vi "Initialize.vi"(8 "error in":errorcluster, 11 "Plugin in":refnum<class "Performanced XNET CAN Logger.lvclass">) -> (0 "error out":errorcluster, 3 "Plugin out":refnum<class "Performanced XNET CAN Logger.lvclass">)   [LabVIEW 2021, in "Performanced XNET CAN Logger.lvlib" / "Performanced XNET CAN Logger.lvclass"]
uses:
  Performanced XNET CAN Logger.lvclass
  C:/Program Files/National Instruments/LabVIEW 2021/vi.lib/FlexLogger/SDK/PluginSDK.lvlibp/PEFClasses/SDK/Plugin/Plugin.lvclass
  Typedef/Def-CAN Port Configuration.ctl
  Typedef/Def-Data Queue Type.ctl
  Typedef/Def-LogSpec.ctl
  Typedef/Def-Executor Command.ctl
  ForFLPlugin/Def-ExecutorConfigurations.ctl
  Performanced XNET CAN Logger.lvclass/Performanced XNET CAN Logger.ctl
  <vilib>/FlexLogger/SDK/PluginSDK.lvlibp/PEFClasses/SDK/Processing Element/Timing Parameters.ctl
  <vilib>/FlexLogger/SDK/PluginSDK.lvlibp/PEFClasses/SDK/Processing Element/Timing Method.ctl
  SubVIs/Global Variables.vi
  <vilib>/FlexLogger/SDK/PluginSDK.lvlibp/PEFClasses/SDK/Plugin/ParameterAccess/Read String.vi
  <vilib>/FlexLogger/SDK/PluginSDK.lvlibp/PEFClasses/SDK/Plugin/ParameterAccess/Write String.vi
  <vilib>/FlexLogger/SDK/PluginSDK.lvlibp/PEFClasses/SDK/Plugin/ParameterAccess/Write Command.vi
  <vilib>/FlexLogger/SDK/PluginSDK.lvlibp/PEFClasses/SDK/Plugin/Plugin.lvclass
  XNET-CAN-Signal-Logger.lvlib
  <vilib>/FlexLogger/SDK/PluginSDK.lvlibp/PEFClasses/SDK/Processing Element/Processing Element.lvclass
  C:/Program Files/National Instruments/LabVIEW 2021/vi.lib/FlexLogger/SDK/PluginSDK.lvlibp/PEFClasses/SDK/Processing Element/Processing Element.lvclass
  C:/Users/NI/Desktop/NIO DongZulong FlexLogger XNET/XNET-CAN-Signal-Logger/src/FlexLogger Plugin/Performanced XNET CAN Logger.lvclass
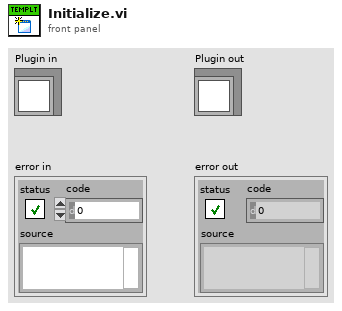
[diagram p1: front panel]
types:
  T1 = typedef "XNET-CAN-Signal-Logger.lvlib/Def-ExecutorConfigurations.ctl" = cluster{"LogSpec":T2, "CAN Configurations":T3[]}
  T2 = typedef "XNET-CAN-Signal-Logger.lvlib/Def-LogSpec.ctl" = cluster{"Log file folder":path, "Log file name":string, "Segment Files":bool, "Segment File Size":i64}
  T3 = typedef "XNET-CAN-Signal-Logger.lvlib/Def-CAN Port Configuration.ctl" = cluster{"CAN Interface":refnum<k21>, "XNET Cluster":refnum<k21>, "#Signals":i32, "Sample Rate (Hz)":dbl}
  T4 = typedef "XNET-CAN-Signal-Logger.lvlib/Def-Executor Command.ctl" = cluster{"Command":string, "Data":variant}
  T5 = typedef "XNET-CAN-Signal-Logger.lvlib/Def-Data Queue Type.ctl" = cluster{"PackageID":i32, "Data":waveform(dbl)[]}
  T6 = typedef "PluginSDK.lvlibp/Processing Element.lvclass/Timing Parameters.ctl" = cluster{"Timing Method":T7, "Timing Period (ms)":i32}
  T7 = typedef "PluginSDK.lvlibp/Processing Element.lvclass/Timing Method.ctl" = enum16{"Periodic", "Immediate", "On Data Ready", "Triggered"}
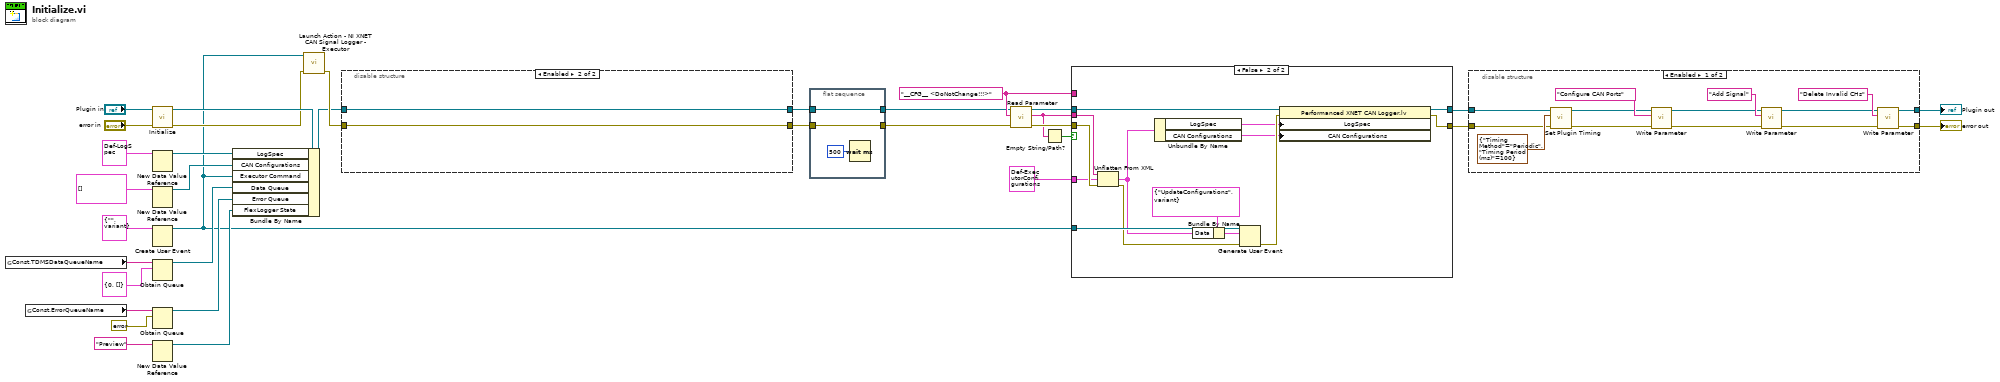
[diagram p0: block diagram]
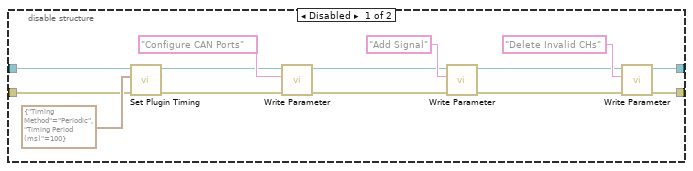
[diagram p3: hidden frame]
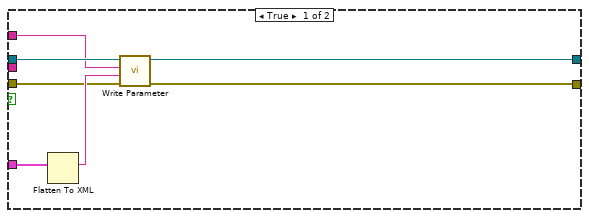
[diagram p4: hidden frame]
diagram:
  w14 = "__CFG__ <DoNotChange!!!>" ("Name")
  n1 = global read "Global Variables.vi" "Const.TDMSDataQueueName"() -> (w29:string)
  n2 = global read "Global Variables.vi" "Const.ErrorQueueName"() -> (w23:string)
  n3 = call-parent "Initialize.vi"("error in (no error)"="error in", "Plugin in"="Plugin in") -> ("error out"=w20:errorcluster, "Plugin out"=w32:refnum<class "Performanced XNET CAN Logger.lvclass">)  [unwired: 8 in]
  n4 = New Data Value Reference(data value=T2 {"Log file folder"=path "C:/Users/NI/Desktop/Data", "Log file name"="Plugin_LogFile_{Year}-{Month}-{Day}-{Hour}-{Minute}-{Second}.tdms", "Segment Files"=FALSE, "Segment File Size"=100} ("LogSpec")) -> (data value reference=w26:refnum<data-value>)  [unwired: 1 in, 1 out]
  n5 = New Data Value Reference(data value=T3[] [] ("Array")) -> (data value reference=w25:refnum<data-value>)  [unwired: 1 in, 1 out]
  n6 = Create User Event(user event datatype=T4 {"Command"="", "Data"=variant} ("Command")) -> (user event=w16:refnum<user-event>)  [unwired: 1 in, 1 out]
  n7 = Obtain Queue(name (unnamed)=w29, element data type=T5 {"PackageID"=0, "Data"=[]} ("Data Queue Type")) -> (queue out=w24:refnum<queue>)  [unwired: 3 in, 2 out]
  n8 = Obtain Queue(name (unnamed)=w23, element data type=errorcluster {"status"=FALSE, "code"=0, "source"=""} ("error in (no error)")) -> (queue out=w22:refnum<queue>)  [unwired: 3 in, 2 out]
  n9 = New Data Value Reference(data value="Preview") -> (data value reference=w18:refnum<data-value>)  [unwired: 1 in, 1 out]
  n10 = Bundle By Name(cluster=w32, "LogSpec"=w26, "CAN Configurations"=w25, "Executor Command"=w16, "Data Queue"=w24, "Error Queue"=w22, "FlexLogger State"=w18) -> (w5:refnum<class "Performanced XNET CAN Logger.lvclass">)
  n11 = call "Launch Action - NI XNET CAN Signal Logger - Executor.vi"("error in (no error)"=w20, "Executor Command"=w16) -> ("error out"=w9:errorcluster)  [unwired: 9 in]
  n12 = disable-structure shown="Enabled" {
    disable-tunnel: w9 -> [w38 w49]
    disable-tunnel: [w37 w49] -> w7
    disable-tunnel: [w36 w50] -> w6
    disable-tunnel: w5 -> [w35 w50]
    frame Disabled {
      n13 = call <vilib>:"Set Plugin Timing.vi"("error in (no error)"=w38, "Timing Parameters"=T6 {"Timing Method"=enum."Periodic", "Timing Period (ms)"=100}, "Plugin in"=w35) -> ("error out"=w40:errorcluster, "Plugin out"=w39:refnum<class "Performanced XNET CAN Logger.lvclass">)  [unwired: 7 in]
      n14 = call-poly <vilib>:"Write Parameter.vi"("error in (no error)"=w40, "Name"="Configure CAN Ports", "Plugin in"=w39) -> ("error out"=w45:errorcluster, "Plugin out"=w46:refnum<class "Performanced XNET CAN Logger.lvclass">)  [unwired: 7 in]
      n15 = call-poly <vilib>:"Write Parameter.vi"("error in (no error)"=w45, "Name"="Add Signal", "Plugin in"=w46) -> ("error out"=w42:errorcluster, "Plugin out"=w43:refnum<class "Performanced XNET CAN Logger.lvclass">)  [unwired: 7 in]
      n16 = call-poly <vilib>:"Write Parameter.vi"("error in (no error)"=w42, "Name"="Delete Invalid CHs", "Plugin in"=w43) -> ("error out"=w37:errorcluster, "Plugin out"=w36:refnum<class "Performanced XNET CAN Logger.lvclass">)  [unwired: 7 in]
    }
    frame Enabled {
    }
  }
  n17 = flat-sequence {
    tunnel: [w53] -> w13
    tunnel: w6 -> [w53]
    tunnel: w7 -> [w52]
    tunnel: [w52] -> w8
    frame #0 {
      n18 = Wait (ms)(milliseconds to wait=u32 500) -> ()  [unwired: 1 out]
    }
  }
  n19 = call-poly <vilib>:"Read Parameter.vi"("error in (no error)"=w8, "Name"=w14, "Plugin in"=w13) -> ("error out"=w15:errorcluster, "Value"=w11:string, "Plugin out"=w17:refnum<class "Performanced XNET CAN Logger.lvclass">)  [unwired: 5 in, 1 out]
  n20 = Empty String/Path?(string/path=w11) -> (empty?=w12:bool)
  n21 = case shown="False" w12 {
    tunnel: [w55 w65] -> w2
    tunnel: w16 -> [_ w72]
    tunnel: [w59 w67] -> w3
    tunnel: w17 -> [w60 w71]
    tunnel: w11 -> [_ w70]
    tunnel: w15 -> [w56 w69]
    tunnel: w14 -> [w58 _]
    tunnel: T1 {"LogSpec"={"Log file folder"=path "C:/Users/NI/Desktop/Data", "Log file name"="Plugin_LogFile_{Year}-{Month}-{Day}-{Hour}-{Minute}-{Second}.tdms", "Segment Files"=FALSE, "Segment File Size"=100}, "CAN Configurations"=[]} ("Executor Configurations") -> [w54 w61]
    frame True {
      n22 = Flatten To XML(6:w54) -> (2:w57:string)
      n23 = call-poly <vilib>:"Write Parameter.vi"("error in (no error)"=w56, "Value"=w57, "Name"=w58, "Plugin in"=w60) -> ("error out"=w55:errorcluster, "Plugin out"=w59:refnum<class "Performanced XNET CAN Logger.lvclass">)  [unwired: 6 in]
    }
    frame False {
      n24 = Unflatten From XML(xml string=w70, type=w61, error in (no error)=w69) -> (value=w64:T1, error out=w68:errorcluster)
      n25 = Unbundle By Name(w64) -> ("LogSpec"=w62:T2, "CAN Configurations"=w63:T3[])
      n26 = Bundle By Name(cluster=T4 {"Command"="UpdateConfigurations", "Data"=variant} ("event data"), "Data"=w64) -> (w73:T4)
      n27 = Generate User Event(user event=w72, event data cluster=w73, error in=w68) -> (error out=w66:errorcluster)  [unwired: 1 in, 1 out]
      n28 = property class="Performanced XNET CAN Logger.lv"(reference=w71, error in=w66, "LogSpec"=w62, "CAN Configurations"=w63) -> (reference out=w67:refnum<class "Performanced XNET CAN Logger.lvclass">, error out=w65:errorcluster)
    }
  }
  n29 = disable-structure shown="Enabled" {
    disable-tunnel: w2 -> [w78 w89]
    disable-tunnel: [w77 w89] -> w1
    disable-tunnel: [w76 w90] -> w4
    disable-tunnel: w3 -> [w75 w90]
    frame Enabled {
      n30 = call <vilib>:"Set Plugin Timing.vi"("error in (no error)"=w78, "Timing Parameters"=T6 {"Timing Method"=enum."Periodic", "Timing Period (ms)"=100}, "Plugin in"=w75) -> ("error out"=w80:errorcluster, "Plugin out"=w79:refnum<class "Performanced XNET CAN Logger.lvclass">)  [unwired: 7 in]
      n31 = call-poly <vilib>:"Write Parameter.vi"("error in (no error)"=w80, "Name"="Configure CAN Ports", "Plugin in"=w79) -> ("error out"=w85:errorcluster, "Plugin out"=w86:refnum<class "Performanced XNET CAN Logger.lvclass">)  [unwired: 7 in]
      n32 = call-poly <vilib>:"Write Parameter.vi"("error in (no error)"=w85, "Name"="Add Signal", "Plugin in"=w86) -> ("error out"=w82:errorcluster, "Plugin out"=w83:refnum<class "Performanced XNET CAN Logger.lvclass">)  [unwired: 7 in]
      n33 = call-poly <vilib>:"Write Parameter.vi"("error in (no error)"=w82, "Name"="Delete Invalid CHs", "Plugin in"=w83) -> ("error out"=w77:errorcluster, "Plugin out"=w76:refnum<class "Performanced XNET CAN Logger.lvclass">)  [unwired: 7 in]
    }
    frame Disabled {
    }
  }
  "error out" <- w1
  "Plugin out" <- w4
